vi "Match Source and Sink Terminals.vi"(8 "error in (no error)":errorcluster, 9 "Node Terminals":refnum<vi>[](array[refnum]), 10 "Node Sources?":bool, 11 "Available Non-Nodes in":T1[](array[typedef])) -> (0 "error out":errorcluster, 2 "Any Changes?":bool, 3 "Available Non-Nodes out":T1[](array[typedef]))   [LabVIEW 2016]
uses:
  <resource>/dialog/QuickDrop/plugins/_WireMultipleSupport/Available Non-Node.ctl
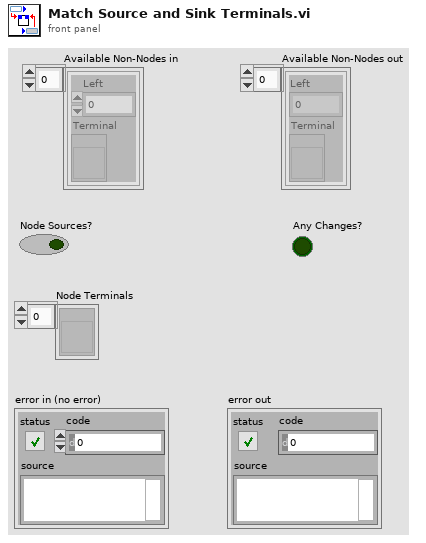
[diagram p1: front panel]
types:
  T1 = typedef "Available Non-Node.ctl" = cluster{"Left":i32, "Terminal":refnum<vi>}
  T2 = cluster{"Top":i32, "Terminal":refnum<vi>, "Data Type":variant}
  T3 = cluster{"Top":i32, "Terminal":refnum<vi>, "Data Type":variant}[]
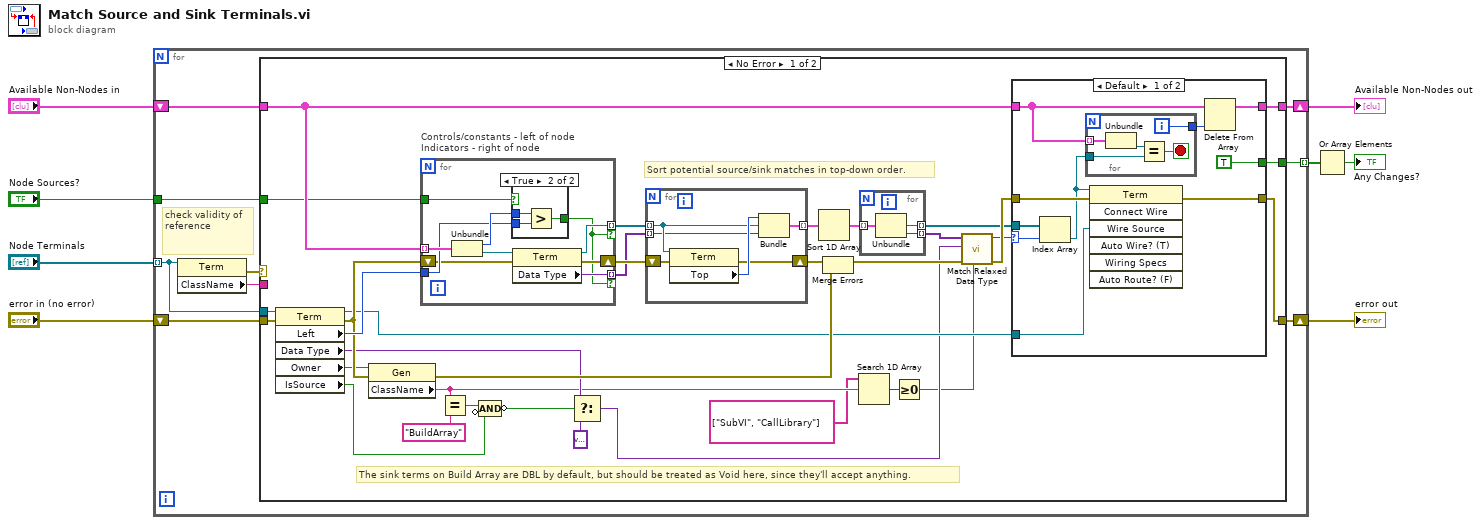
[diagram p0: block diagram]
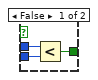
[diagram p3: hidden frame]
diagram:
  n1 = for {
    tunnel: "Node Terminals" -> [w10] mode=indexing
    shift-right: [w15] -> w5
    shift-left: "error in (no error)" -> [w9]
    shift-right: [w16] -> w3
    shift-left: "Available Non-Nodes in" -> [w17]
    tunnel: [w14] -> w4 mode=indexing
    tunnel: "Node Sources?" -> [w11]
    # "check validity of reference"
    n2 = property class="Term"(reference=w10) -> (error out=w12:errorcluster, "ClassName"=w13:string)  [unwired: 1 in, 1 out]
    n3 = case shown="No Error" w12 {
      tunnel: w9 -> [w51 w95]
      tunnel: w17 -> [w49 w94]
      tunnel: [w48 w94] -> w16
      tunnel: [w47 w95] -> w15
      tunnel: [w46 _] -> w14
      tunnel: w10 -> [w43 _]
      tunnel: w13 -> [_ _]
      tunnel: w11 -> [w42 _]
      frame No Error {
        # "The sink terms on Build Array are DBL by default, but should be treated as Void here, since they'll accept anything."
        # "Sort potential source/sink matches in top-down order."
        n4 = property class="Term"(reference=w43, error in=w51) -> (reference out=w26:refnum<vi>, error out=w32:errorcluster, "Left"=w50:i32, "Data Type"=w24:variant, "Owner"=w31:refnum<vi>, "IsSource"=w28:bool)
        n5 = property class="Gen"(reference=w31, error in=w32) -> (error out=w27:errorcluster, "ClassName"=w21:string)  [unwired: 1 out]
        n6 = for "Controls/constants - left of node\nIndicators - right of node" {
          tunnel: w49 -> [w87] mode=indexing
          tunnel: [w86] -> w40 mode=indexing if=w79
          tunnel: w50 -> [w84]
          shift-right: [w82] -> w41
          shift-left: w32 -> [w83]
          tunnel: [w81] -> w39 mode=indexing if=w79
          tunnel: w42 -> [w80]
          n7 = Unbundle(w87) -> ("Left"=w85:i32, "Terminal"=w78:refnum<vi>)
          n8 = case shown="True" w80 {
            tunnel: w85 -> [w90 w92]
            tunnel: w84 -> [w89 w93]
            tunnel: [w88 w91] -> w79
            frame False {
              n9 = Less?(x=w90, y=w89) -> (x < y?=w88:bool)
            }
            frame True {
              n10 = Greater?(x=w92, y=w93) -> (0:w91:bool)
            }
          }
          n11 = property class="Term"(reference=w78, error in=w83) -> (reference out=w81:refnum<vi>, error out=w82:errorcluster, "Data Type"=w86:variant)
        }
        n12 = Equal?(x=w21, y="BuildArray") -> (x = y?=w29:bool)
        n13 = Compound Arithmetic op=AND(w29, invert w28) -> (invert w25:bool)
        n14 = Select(t=w24, s=w25, f=variant) -> (s? t:f=w22:variant)
        n15 = for {
          tunnel: w40 -> [w56] mode=indexing
          tunnel: w39 -> [w57] mode=indexing
          shift-right: [w58] -> w38
          shift-left: w41 -> [w60]
          tunnel: [w55] -> w37 mode=indexing
          n16 = property class="Term"(reference=w57, error in=w60) -> (error out=w58:errorcluster, "Top"=w59:i32)  [unwired: 1 out]
          n17 = Bundle("Top"=w59, "Terminal"=w57, "Data Type"=w56) -> (w55:T2)  [unwired: 1 in]
        }
        n18 = Sort 1D Array(array=w37) -> (sorted array=w36:T3)
        n19 = Merge Errors(w38, w27) -> (w33:errorcluster)
        n20 = Search 1D Array(1D array=string[] ["SubVI", "CallLibrary"], element=w21) -> (index of element=w19:i32)  [unwired: 1 in]
        n21 = for {
          tunnel: w36 -> [w54] mode=indexing
          tunnel: [w53] -> w35 mode=indexing
          tunnel: [w52] -> w34 mode=indexing
          n22 = Unbundle(w54) -> ("Terminal"=w53:refnum<vi>, "Data Type"=w52:variant)  [unwired: 1 out]
        }
        n23 = Greater Or Equal To 0?(x=w19) -> (x >= 0?=w18:bool)
        n24 = call <resource>:"Match Relaxed Data Type.vi"("Invalid Void Terms?"=w18, "error in (no error)"=w33, "Data Type to Match"=w22, "Array of Data Types"=w34) -> ("error out"=w45:errorcluster, "Matched Index"=w44:i32)  [unwired: 6 in]
        n25 = case shown="Default" w44 {
          selector: w44 -> [w61 _]
          tunnel: w45 -> [w70 w77]
          tunnel: [w62 w77] -> w47
          tunnel: [TRUE _] -> w46
          tunnel: w49 -> [w66 w76]
          tunnel: [w65 w76] -> w48
          tunnel: w35 -> [w68 _]
          tunnel: w26 -> [w63 _]
          frame Default {
            n26 = Index Array(array=w68, index=w61) -> (element=w67:refnum<vi>)
            n27 = for {
              tunnel: w66 -> [w75] mode=indexing
              tunnel: w67 -> [w73]
              tunnel: [w71] -> w64
              i -> [w71]
              stop <- w72 stop-if-true
              n28 = Unbundle(w75) -> ("Terminal"=w74:refnum<vi>)  [unwired: 1 out]
              n29 = Equal?(x=w74, y=w73) -> (x = y?=w72:bool)
            }
            n30 = invoke class="Term" method="Connect Wire"(reference=w67, error in=w70, "Wire Source"=w63) -> (error out=w62:errorcluster)  [unwired: 4 in, 6 out]
            n31 = Delete From Array(array=w66, index=w64) -> (array with subset deleted=w65:T1[])  [unwired: 1 in, 1 out]
          }
          frame -1 {
            # "No comparable data type found for this item.\nDon't try to wire it up."
          }
        }
      }
      frame Error {
        # "Sometimes previous wiring operations can cause old terminals to disappear. The best example of this is an Add function that loses its Pacman error terminals based on a non-waveform type being wired to one of its inputs. If a terminal is found that returns an error (when it previously did not), then ignore it."
      }
    }
  }
  "error out" <- w5
  "Available Non-Nodes out" <- w3
  n32 = Or Array Elements(Boolean array=w4) -> (logical OR=→"Any Changes?":bool)
